vi "Set Ref Level (dBm).vi"(8 "error in (no error)":errorcluster caption="entrée d'erreur (pas d'erreur)", 10 "Ref Level (dBm)":dbl=10.0 min=-170.0 max=50.0 step=0.1, 11 "Class Spectrum Analyser (Default) en entrée":refnum<class "Class Spectrum Analyser (Default).lvclass">) -> (0 "error out":errorcluster caption="sortie d'erreur", 3 "Class Spectrum Analyser (Default) en sortie":refnum<class "Class Spectrum Analyser (Default).lvclass">)   [LabVIEW 2020, in "Library Instrument & Equipement.lvlib" / "Library Spectrum Analyser.lvlib" / "Class Spectrum Analyser (Default).lvclass"]
uses:
  Class Spectrum Analyser (Default).lvclass
  Class Spectrum Analyser (Default).lvclass/Class Spectrum Analyser (Default).ctl
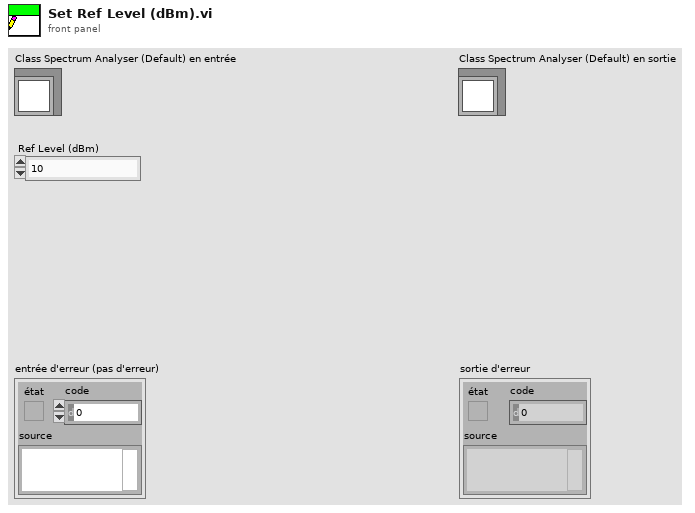
[diagram p1: front panel]
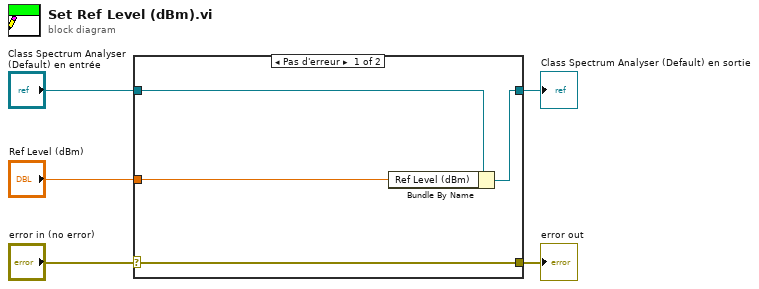
[diagram p0: block diagram]
diagram:
  n1 = case shown="Pas d'erreur" "error in (no error)" {
    selector: "error in (no error)" -> [w9 w10]
    tunnel: [w9 w10] -> w4
    tunnel: [w7 w11] -> w2
    tunnel: "Class Spectrum Analyser (Default) en entrée" -> [w8 w11]
    tunnel: "Ref Level (dBm)" -> [w6 _]
    frame No Error {
      n2 = Bundle By Name(cluster=w8, "Ref Level (dBm)"=w6) -> (w7:refnum<class "Class Spectrum Analyser (Default).lvclass">)
    }
    frame Error {
    }
  }
  "error out" <- w4
  "Class Spectrum Analyser (Default) en sortie" <- w2
